vi "11_Histogram2D.vi"(8 "error in (no error)":errorcluster) -> (0 "error out":errorcluster)   [LabVIEW 2014]
uses:
  SwabianInstruments.TimeTagger
panel:
  in  "binwidth":i64=1
  in  "n_bins_2":i32=300
  in  "n_bins_1":i32=400
  out "Histogram2D":i32[][](graph)
  # "Histogram2D. Each pixel represent a bin with the bin value as color.\nEach bin corresponds to specific time delay between each stop signal and the start signal.\nSo the bin coordinate to de incremented is calculated as (stop1-start, stop2-start) rounded to \nthe corersponding bin boundary.\n\nIn this example we use internal signal generator as start, stop1 and stop2 signals we expect to see \na small, jitter limited, Gaussian like spot located at the position that is generally offset from zero due to small delay \ndifference between channels."
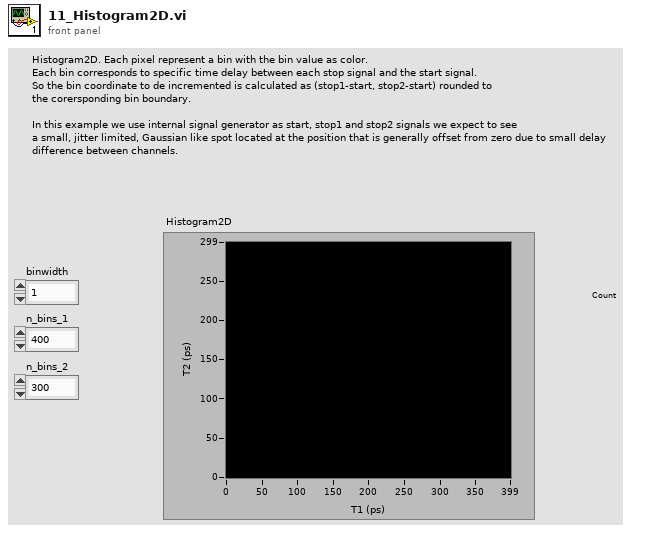
[diagram p1: front panel]
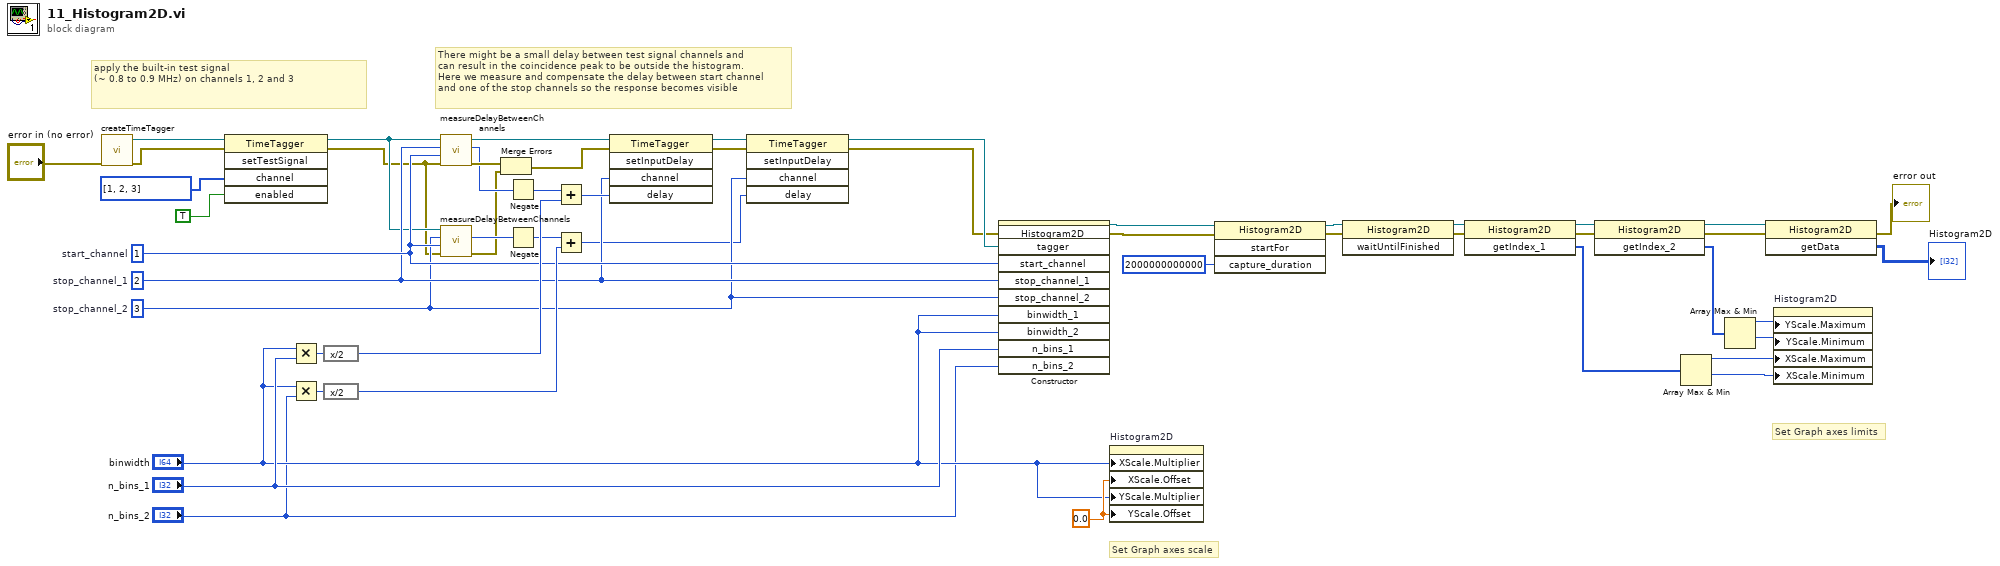
[diagram p0: block diagram]
diagram:
  w44 = 0.0 ("X Scale.Offset and Multiplier:Offset")
  w17 = 3  # stop_channel_2
  w18 = 2  # stop_channel_1
  w19 = 1  # start_channel
  # "There might be a small delay between test signal channels and \ncan result in the coincidence peak to be outside the histogram.\nHere we measure and compensate the delay between start channel\nand one of the stop channels so the response becomes visible"
  # "Set Graph axes limits"
  # "Set Graph axes scale"
  # "apply the built-in test signal\n(~ 0.8 to 0.9 MHz) on channels 1, 2 and 3"
  n1 = call "createTimeTagger.vi"("error in (no error)"="error in (no error)") -> ("error out"=w36:errorcluster, "TimeTagger ref out"=w37:refnum<k24>)  [unwired: 9 in]
  n2 = invoke class="TimeTagger" method="setTestSignal"(reference=w37, error in=w36, "channel"=i32[] [1, 2, 3], "enabled"=TRUE) -> (reference out=w15:refnum<k24>, error out=w3:errorcluster)  [unwired: 1 in, 3 out]
  n3 = Multiply(x="binwidth", y="n_bins_1") -> (x*y=w28:i64)
  n4 = Multiply(x="binwidth", y="n_bins_2") -> (x*y=w27:i64)
  n5 = expression code="x/2"(w28) -> (w26:i64)
  n6 = expression code="x/2"(w27) -> (w25:i64)
  n7 = call "measureDelayBetweenChannels.vi"("error in (no error)"=w3, "channel_2"=w19, "channel_1"=w18, "TimeTagger ref in"=w15) -> ("error out"=w34:errorcluster, "measured delay, ps"=w33:i64, "TimeTagger ref out"=w35:refnum<k24>)  [unwired: 5 in]
  n8 = call "measureDelayBetweenChannels.vi"("error in (no error)"=w3, "channel_2"=w19, "channel_1"=w17, "TimeTagger ref in"=w15) -> ("error out"=w1:errorcluster, "measured delay, ps"=w23:i64)  [unwired: 5 in, 1 out]
  n9 = Merge Errors(w34, w1) -> (w2:errorcluster)
  n10 = Negate(x=w33) -> (-x=w32:i64)
  n11 = Negate(x=w23) -> (-x=w22:i64)
  n12 = Add(x=w32, y=w26) -> (x+y=w24:i64)
  n13 = Add(x=w22, y=w25) -> (x+y=w16:i64)
  n14 = invoke class="TimeTagger" method="setInputDelay"(reference=w35, error in=w2, "channel"=w18, "delay"=w24) -> (reference out=w21:refnum<k24>, error out=w20:errorcluster)  [unwired: 1 in, 3 out]
  n15 = invoke class="TimeTagger" method="setInputDelay"(reference=w21, error in=w20, "channel"=w17, "delay"=w16) -> (reference out=w14:refnum<k24>, error out=w13:errorcluster)  [unwired: 1 in, 3 out]
  n16 = constructor class="Histogram2D"(error in=w13, "tagger"=w14, "start_channel"=w19, "stop_channel_1"=w18, "stop_channel_2"=w17, "binwidth_1"="binwidth", "binwidth_2"="binwidth", "n_bins_1"="n_bins_1", "n_bins_2"="n_bins_2") -> (reference out=w12:refnum<k24>, error out=w11:errorcluster)  [unwired: 2 in, 9 out]
  n17 = property on="Histogram2D" class="IntGraph (strict)"("XScale.Multiplier"="binwidth", "XScale.Offset"=w44, "YScale.Multiplier"="binwidth", "YScale.Offset"=w44) -> ()  [unwired: 2 in, 2 out]
  n18 = invoke class="Histogram2D" method="startFor"(reference=w12, error in=w11, "capture_duration"=i64 2000000000000) -> (reference out=w9:refnum<k24>, error out=w6:errorcluster)  [unwired: 1 in, 2 out]
  n19 = invoke class="Histogram2D" method="waitUntilFinished"(reference=w9, error in=w6) -> (reference out=w8:refnum<k24>, error out=w7:errorcluster)  [unwired: 1 in, 1 out]
  n20 = invoke class="Histogram2D" method="getIndex_1"(reference=w8, error in=w7) -> (reference out=w48:refnum<k24>, error out=w47:errorcluster, "getIndex_1"=w43:i64[])  [unwired: 1 in]
  n21 = invoke class="Histogram2D" method="getIndex_2"(reference=w48, error in=w47) -> (reference out=w45:refnum<k24>, error out=w46:errorcluster, "getIndex_2"=w42:i64[])  [unwired: 1 in]
  n22 = Array Max & Min(array=w43) -> (max value=w39:i64, min value=w38:i64)  [unwired: 2 out]
  n23 = Array Max & Min(array=w42) -> (max value=w41:i64, min value=w40:i64)  [unwired: 2 out]
  n24 = invoke class="Histogram2D" method="getData"(reference=w45, error in=w46) -> (error out=→"error out":errorcluster, "getData"=→"Histogram2D":i32[][])  [unwired: 1 in, 1 out]
  n25 = property on="Histogram2D" class="IntGraph (strict)"("YScale.Maximum"=w41, "YScale.Minimum"=w40, "XScale.Maximum"=w39, "XScale.Minimum"=w38) -> ()  [unwired: 2 in, 2 out]
